vi "Initialize.vi"(8 "error in (no error)":errorcluster, 11 "Muon Detector in":refnum<class "Muon Detector.lvclass">) -> (0 "error out":errorcluster, 3 "Muon Detector out":refnum<class "Muon Detector.lvclass">)   [LabVIEW 2019, in "Muon Detector.lvclass"]
uses:
  Muon Detector.lvclass
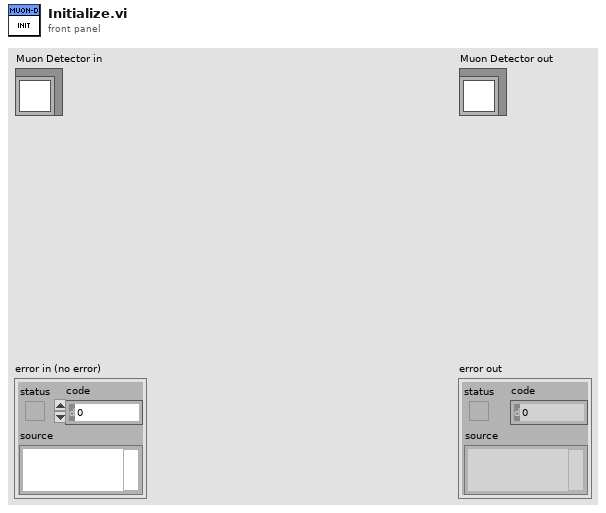
[diagram p1: front panel]
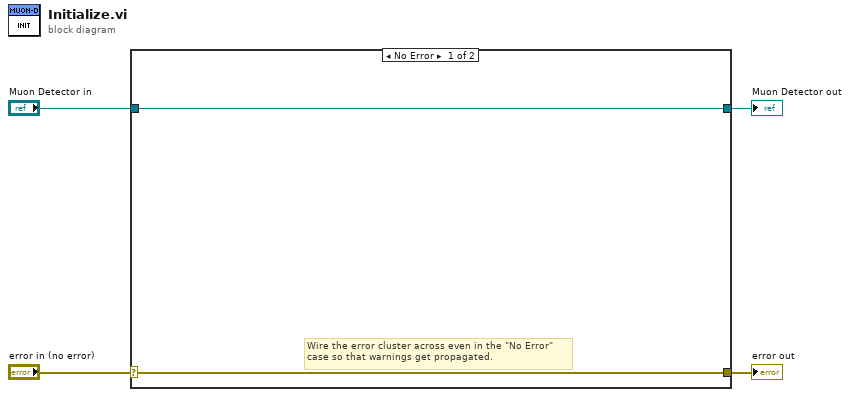
[diagram p0: block diagram]
diagram:
  n1 = case shown="No Error" "error in (no error)" {
    selector: "error in (no error)" -> [w5 w8]
    tunnel: [w5 w8] -> w3
    tunnel: [w6 w7] -> w1
    tunnel: "Muon Detector in" -> [w6 w7]
    frame No Error {
      # "Wire the error cluster across even in the \"No Error\"\ncase so that warnings get propagated."
    }
    frame Error {
    }
  }
  "error out" <- w3
  "Muon Detector out" <- w1
